vi "hp83623a close.vi"(8 "error in (no error)":errorcluster, 11 "hp83623a Settings In":T1={"Frequency (Hz)"="20000000", "Power (dBm)"="0", "Enabled"=TRUE, "initialized"=FALSE, "RF Output On/Off"=TRUE, "External Trigger?"=FALSE, "VISA Session"="GPIB0::3::INSTR", "Generator Name"="Generator"}) -> (0 "error out":errorcluster)   [LabVIEW 2012, in "HP83623A_RF_Generator.lvclass"]
uses:
  HP83623A_RF_Generator.lvclass
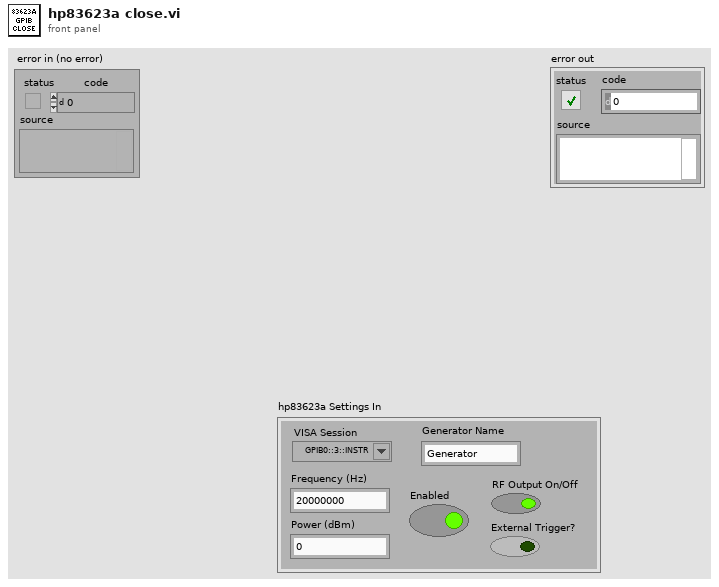
[diagram p1: front panel]
types:
  T1 = cluster{"Frequency (Hz)":string, "Power (dBm)":string, "Enabled":bool, "initialized":bool, "RF Output On/Off":bool, "External Trigger?":bool, "VISA Session":refnum<visa-resource-name>, "Generator Name":string}
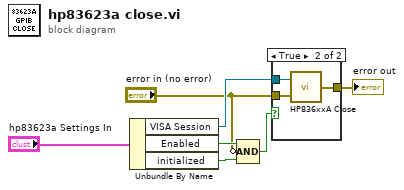
[diagram p0: block diagram]
diagram:
  n1 = Unbundle By Name("hp83623a Settings In") -> ("VISA Session"=w6:refnum<visa-resource-name>, "Enabled"=w4:bool, "initialized"=w2:bool)
  n2 = Compound Arithmetic op=AND(w4, invert "error in (no error)", w2) -> (w1:bool)
  n3 = case shown="True" w1 {
    tunnel: w6 -> [_ w11]
    tunnel: "error in (no error)" -> [w8 w10]
    tunnel: [w8 w9] -> w5
    frame False {
    }
    frame True {
      n4 = call "HP836xxA Close.vi"("error in (no error)"=w10, "VISA session"=w11) -> ("error out"=w9:errorcluster)
    }
  }
  "error out" <- w5
